vi "Test Read and Move.vi"(7 "Stop Button":bool, 10 "Auto Feed Control":T1) -> ()   [LabVIEW 2013]
doc: "This VI tests reading positions from all three axes simultaneously, and sending move commands to the\naxes using the NI Motion Assistant Move Hander."
uses:
  <vilib>/MotionAssistant/MotionAssistant.llb/Move Constraints.ctl
  <vilib>/MotionAssistant/MotionAssistant.llb/Velocity Profile Type Enum.ctl
  Controls/axis_indicator_cluster.ctl
  Controls/auto_feed_control_cluster.ctl
  <vilib>/MotionAssistant/MotionAssistant.llb/Straight Line Move Properties.ctl
  <vilib>/MotionAssistant/MotionAssistant.llb/Straight Line Dimension Enum.ctl
  <vilib>/MotionAssistant/MotionAssistant.llb/Straight Line Move Mode Enum.ctl
  <vilib>/MotionAssistant/MotionAssistant.llb/Coordinate Point.ctl
  Controls/PWM_data_cluster.ctl
  Controls/table_axis_enum.ctl
  Controls/PWM_state_enum.ctl
  <vilib>/MotionAssistant/MotionAssistant.llb/Profile Calculation Constraint.ctl
  <vilib>/MotionAssistant/MotionAssistant.llb/Array Constraints Spec Type Enum.ctl
  <vilib>/MotionAssistant/MotionAssistant.llb/Move Profile Enum.ctl
  <vilib>/MotionAssistant/MotionAssistant.llb/Open Straight Line Move Handle.vi
  <vilib>/MotionAssistant/MotionAssistant.llb/Close Straight Line Move Handle.vi
  <vilib>/MotionAssistant/MotionAssistant.llb/Set Straight Line Move Properties.vi
  <vilib>/MotionAssistant/MotionAssistant.llb/Get Straight Line Move Profile.vi
panel:
  out "Axis Inds.":T2 caption="Axis Indicators"
  in  "Move Constraints":T3={"Velocity Profile Type"=enum."S Curve", "Max Velocity"=2.0, "Max Acceleration"=1.0, "Max Deceleration"=1.0, "Max Jerk"=2.0, "Initial Velocity"=0.0, "Final Velocity"=0.0} {"Final Velocity" format="%#.6g"; "Initial Velocity" format="%#.6g"; "Max Jerk" format="%#.6g"; "Max Deceleration" format="%#.6g"; "Max Acceleration" format="%#.6g"; "Max Velocity" format="%#.6g"}
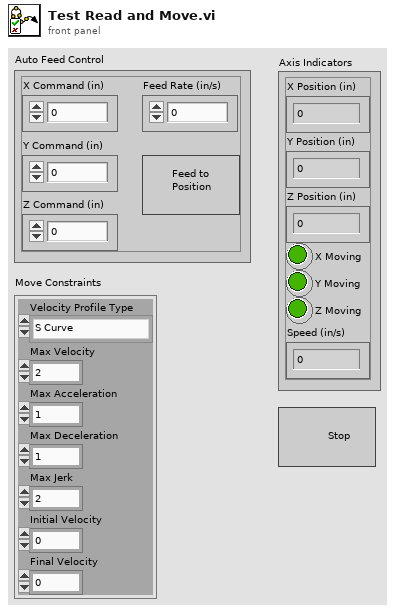
[diagram p1: front panel]
types:
  T1 = typedef "auto_feed_control_cluster.ctl" = cluster{"Feed Rate (in/s)":dbl, "X Command (in)":dbl, "Y Command (in)":dbl, "Z Command (in)":dbl, "feed to pos":bool}
  T2 = typedef "axis_indicator_cluster.ctl" = cluster{"X Position (in)":dbl, "Y Position (in)":dbl, "Z Position (in)":dbl, "X Moving":bool, "Y Moving":bool, "Z Moving":bool, "Speed (in/s)":dbl}
  T3 = typedef "Move Constraints.ctl" = cluster{"Velocity Profile Type":T4, "Max Velocity":dbl, "Max Acceleration":dbl, "Max Deceleration":dbl, "Max Jerk":dbl, "Initial Velocity":dbl, "Final Velocity":dbl}
  T4 = typedef "Velocity Profile Type Enum.ctl" = enum32{"Trapezoidal", "S Curve"}
  T5 = typedef "PWM_data_cluster.ctl" = cluster{"frequency":dbl, "Duty Cycle (%)":dbl, "Axis Enum":T6, "Function Enum":T7}
  T6 = typedef "table_axis_enum.ctl" = enum16{"X-axis", "Y-axis", "Z-axis", "W-axis"}
  T7 = typedef "PWM_state_enum.ctl" = enum16{"Initialize", "SetAxisSpeed", "StopAxis", "StopAll", "Shutdown"}
  T8 = typedef "Straight Line Move Properties.ctl" = cluster{"Dimension":T9, "Move Mode":T10, "Position Mode - End Point":T11, "Velocity Mode - Travel Time (sec)":dbl}
  T9 = typedef "Straight Line Dimension Enum.ctl" = enum16{"1-Dimension", "2-Dimension", "3-Dimension"}
  T10 = typedef "Straight Line Move Mode Enum.ctl" = enum32{" Position Mode", "Velocity Mode"}
  T11 = typedef "Coordinate Point.ctl" = cluster{"X":dbl, "Y":dbl, "Z":dbl}
  T12 = cluster{"Straight Line Move Properties":T8, "Start Point":T11}
  T13 = typedef "Straight Line Move Handle.ctl" = cluster{"Straight Line Move Enum":T14, "Move Handle":i32}
  T14 = typedef "Straight Line Move Enum.ctl" = enum16{"Straight Line Move"}
  T15 = typedef "Move Profile Enum.ctl" = enum16{"Velocity Profile", "Acceleration Profile", "Position Profile"}
  T16 = typedef "Profile Calculation Constraint.ctl" = cluster{"Constraint Type":T17, "Constraint Value":dbl}
  T17 = typedef "Array Constraints Spec Type Enum.ctl" = enum16{"Array Size", "Sampling Time"}
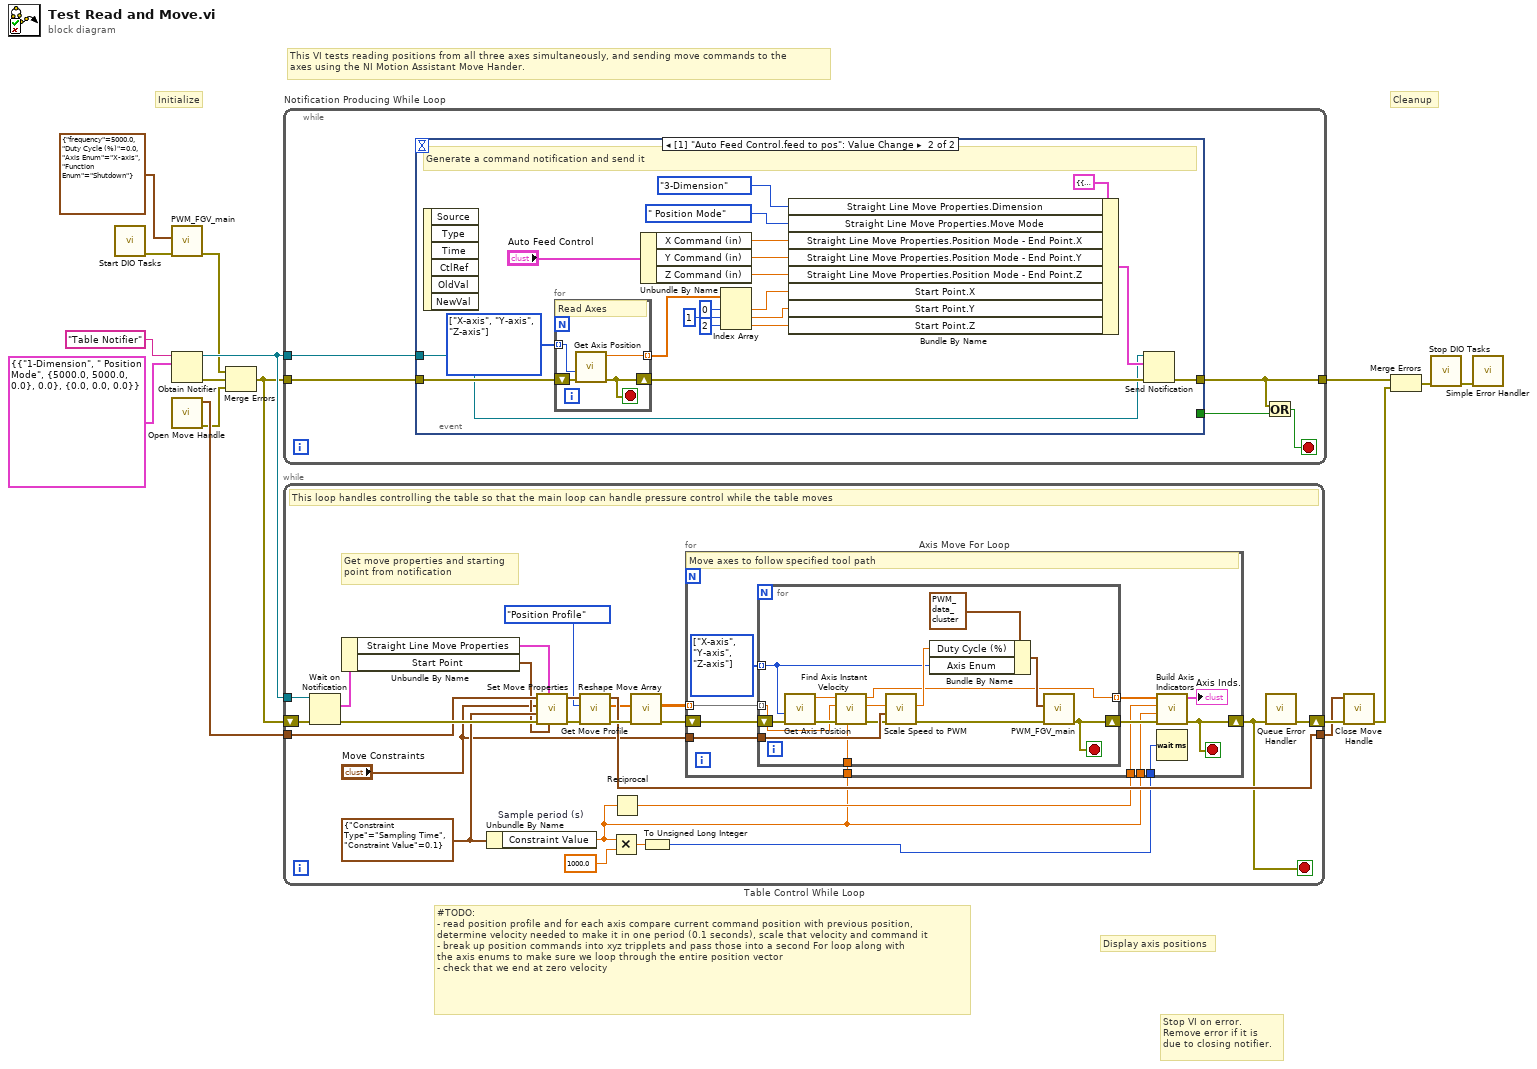
[diagram p0: block diagram]
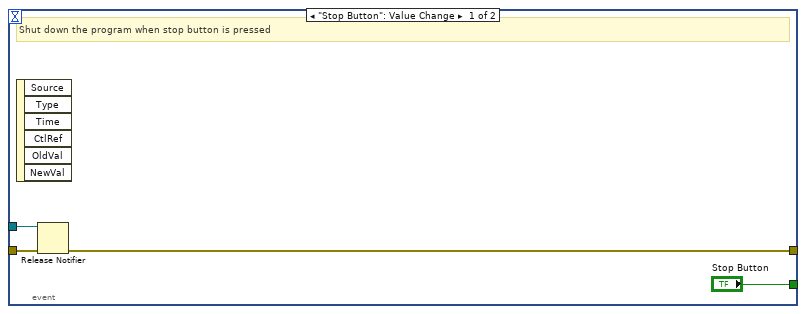
[diagram p2: hidden frame]
diagram:
  # "Stop VI on error.\nRemove error if it is\ndue to closing notifier."
  # "Display axis positions"
  # "#TODO:\n- read position profile and for each axis compare current command position with previous position,\ndetermine velocity needed to make it in one period (0.1 seconds), scale that velocity and command it\n- break up position commands into xyz tripplets and pass those into a second For loop along with\nthe axis enums to make sure we loop through the entire position vector\n- check that we end at zero velocity"
  # "Initialize"
  # "Cleanup"
  # "This VI tests reading positions from all three axes simultaneously, and sending move commands to the\naxes using the NI Motion Assistant Move Hander."
  n1 = call "Start DIO Tasks.vi"() -> ("error out"=w3:errorcluster)  [unwired: 11 in]
  n2 = call "PWM_FGV_main.vi"("Error In"=w3, "PWM FGV Data"=T5 {"frequency"=5000.0, "Duty Cycle (%)"=0.0, "Axis Enum"=enum."X-axis", "Function Enum"=enum."Shutdown"}) -> ("Error Out"=w8:errorcluster)  [unwired: 9 in]
  n3 = Obtain Notifier(name (unnamed)="Table Notifier", notification data type=T12 {"Straight Line Move Properties"={"Dimension"=enum."1-Dimension", "Move Mode"=enum." Position Mode", "Position Mode - End Point"={"X"=5000.0, "Y"=5000.0, "Z"=0.0}, "Velocity Mode - Travel Time (sec)"=0.0}, "Start Point"={"X"=0.0, "Y"=0.0, "Z"=0.0}}) -> (notifier out=w13:refnum<notifier>, error out=w12:errorcluster)  [unwired: 2 in, 1 out]
  n4 = call-poly <vilib>:"Open Move Handle.vi"() -> ("error out"=w11:errorcluster, "Straight Line Move Handle"=w16:T13)  [unwired: 9 in]
  n5 = Merge Errors(w8, w12, w11) -> (w10:errorcluster)
  n6 = while "Notification Producing While Loop" {
    tunnel: w13 -> [w17]
    tunnel: w10 -> [w18]
    tunnel: [w20] -> w4
    stop <- w21 stop-if-true
    n7 = event shown="[1] \"Auto Feed Control.feed to pos\": Value Change" {
      selector: _ -> [_ _]
      dyn-events: _ -> [_ _]
      timeout: _ -> [_ _]
      tunnel: ["Stop Button" _] -> w19
      tunnel: [w24 w45] -> w20
      tunnel: w18 -> [w23 w29]
      tunnel: w17 -> [w22 w28]
      event "Stop Button": Value Change {
        # "Shut down the program when stop button is pressed"
        n8 = event-data() -> ()  [unwired: 1 in, 6 out]
        n9 = Release Notifier(notifier=w22, error in (no error)=w23) -> (error out=w24:errorcluster)  [unwired: 1 in, 2 out]
      }
      event Value Change {
        w38 = T6[] [enum."X-axis", enum."Y-axis", enum."Z-axis"] items=["X-axis", "Y-axis", "Z-axis", "W-axis"]
        # "Generate a command notification and send it"
        n10 = event-data() -> ()  [unwired: 1 in, 6 out]
        n11 = for "Read Axes" {
          shift-right: [w48] -> w39
          shift-left: w29 -> [w49]
          tunnel: w38 -> [w47] mode=indexing
          tunnel: [w46] -> w37 mode=indexing
          stop <- w48 stop-if-true
          # "Read Axes"
          n12 = call "Get Axis Position.vi"("Error In"=w49, "Axis Enum"=w47) -> ("Error Out"=w48:errorcluster, "Axis Inches"=w46:dbl)  [unwired: 6 in, 2 out]
        }
        n13 = Unbundle By Name("Auto Feed Control") -> ("X Command (in)"=w42:dbl, "Y Command (in)"=w41:dbl, "Z Command (in)"=w40:dbl)
        n14 = Index Array(array=w37, index #1=0 ("index"), index #2=1 ("index"), index #3=2 ("index")) -> (element #1=w36:dbl, element #2=w34:dbl, element #3=w35:dbl)
        n15 = Bundle By Name(cluster=T12 {"Straight Line Move Properties"={"Dimension"=enum."1-Dimension", "Move Mode"=enum." Position Mode", "Position Mode - End Point"={"X"=0.0, "Y"=0.0, "Z"=0.0}, "Velocity Mode - Travel Time (sec)"=0.0}, "Start Point"={"X"=0.0, "Y"=0.0, "Z"=0.0}} ("notification"), "Straight Line Move Properties.Dimension"=Straight_Line_Dimension_Enum."3-Dimension", "Straight Line Move Properties.Move Mode"=Straight_Line_Move_Mode_Enum." Position Mode", "Straight Line Move Properties.Position Mode - End Point.X"=w42, "Straight Line Move Properties.Position Mode - End Point.Y"=w41, "Straight Line Move Properties.Position Mode - End Point.Z"=w40, "Start Point.X"=w36, "Start Point.Y"=w34, "Start Point.Z"=w35) -> (w30:T12)
        n16 = Send Notification(notification=w30, notifier=w28, error in (no error)=w39) -> (error out=w45:errorcluster)  [unwired: 1 out]
      }
    }
    n17 = Or(x=w20, y=w19) -> (x .or. y?=w21:bool)
  }
  n18 = while "Table Control While Loop" {
    shift-right: [w72] -> w7
    shift-left: w10 -> [w71]
    tunnel: w13 -> [w70]
    tunnel: w16 -> [w65]
    tunnel: [w57] -> w5
    stop <- w52 stop-if-true
    w63 = T16 {"Constraint Type"=enum."Sampling Time", "Constraint Value"=0.1} ("Profile Calculation Constraint")
    # "Get move properties and starting\npoint from notification"
    # "This loop handles controlling the table so that the main loop can handle pressure control while the table moves"
    n19 = Wait on Notification(notifier=w70, error in (no error)=w71) -> (notification=w60:T12, error out=w66:errorcluster)  [unwired: 2 in, 2 out]
    n20 = Unbundle By Name(w60) -> ("Straight Line Move Properties"=w59:T8, "Start Point"=w58:T11)
    n21 = Unbundle By Name "Sample period (s)"(w63) -> ("Constraint Value"=w54:dbl)
    n22 = call-poly <vilib>:"Set Move Properties.vi"("Start Point"=w58, "Straight Line Move Properties"=w59, "error in"=w66, "Profile Calculation Constraint"=w63, "Move Constraints"="Move Constraints", "Straight Line Move Handle In"=w65) -> ("error out"=w69:errorcluster, "Straight Line Move Handle Out"=w68:T13)  [unwired: 3 in]
    n23 = call-poly <vilib>:"Get Move Profile.vi"("error in"=w69, "Profile Type"=Move_Profile_Enum."Position Profile", "Straight Line Move Handle In"=w68) -> ("error out"=w67:errorcluster, "Profile"=w51:dbl[], "Straight Line Move Handle Out"=w57:T13)  [unwired: 3 in, 2 out]
    n24 = Multiply(x=w54, y=1000.0) -> (x*y=w62:dbl)
    n25 = Reciprocal(x=w54) -> (1/x=w55:dbl)
    n26 = call "Reshape Move Array.vi"("Profile in"=w51) -> ("Profile out"=w50:dbl[][])  [unwired: 10 in]
    n27 = To Unsigned Long Integer(number=w62) -> (unsigned 32bit integer=w53:u32)
    n28 = for "Axis Move For Loop" {
      shift-right: [w80] -> w52
      shift-left: w67 -> [w83]
      tunnel: "Move Constraints" -> [w84]
      tunnel: w50 -> [w82] mode=indexing
      tunnel: w54 -> [w81]
      tunnel: w55 -> [w75]
      tunnel: w54 -> [w76]
      tunnel: w53 -> [w77]
      stop <- w80 stop-if-true
      w74 = T6[] [enum."X-axis", enum."Y-axis", enum."Z-axis"] items=["X-axis", "Y-axis", "Z-axis", "W-axis"]
      # "Move axes to follow specified tool path"
      n29 = for {
        tunnel: w84 -> [w99]
        tunnel: w82 -> [w90] mode=indexing
        tunnel: w81 -> [w88]
        shift-right: [w86] -> w79
        shift-left: w83 -> [w95]
        tunnel: w74 -> [w87] mode=indexing
        tunnel: [w85] -> w73 mode=indexing
        stop <- w86 stop-if-true
        n30 = call "Get Axis Position.vi"("Error In"=w95, "Axis Enum"=w87) -> ("Error Out"=w93:errorcluster, "Axis Inches"=w92:dbl)  [unwired: 6 in, 2 out]
        n31 = call "Find Axis Instant Velocity.vi"("Sample Period"=w88, "Error In"=w93, "Desired Position"=w90, "Current Position"=w92) -> ("Error Out"=w89:errorcluster, "Axis Velocity"=w91:dbl, "Current Position out"=w85:dbl)  [unwired: 5 in]
        n32 = call "Scale Speed to PWM.vi"("Error In"=w89, "Move Constraints"=w99, "Desired Speed (in/s)"=w91) -> ("Error Out"=w94:errorcluster, "Motor Duty Cycle"=w96:dbl)  [unwired: 7 in]
        n33 = Bundle By Name(cluster=T5 {"frequency"=5000.0, "Duty Cycle (%)"=0.0, "Axis Enum"=enum."X-axis", "Function Enum"=enum."Shutdown"} ("PWM FGV Data"), "Duty Cycle (%)"=w96, "Axis Enum"=w87) -> (w97:T5)
        n34 = call "PWM_FGV_main.vi"("Error In"=w94, "PWM FGV Data"=w97) -> ("Error Out"=w86:errorcluster)  [unwired: 9 in]
      }
      n35 = call "Build Axis Indicators.vi"("Error In"=w79, "Sample Period"=w76, "Sample Freq."=w75, "Axis Pos."=w73) -> ("Error Out"=w80:errorcluster, "Axis Inds. out"=→"Axis Inds.":T2)  [unwired: 6 in]
      n36 = Wait (ms)(milliseconds to wait=w77) -> ()  [unwired: 1 out]
    }
    n37 = call "Queue Error Handler.vi"("Error In"=w52) -> ("Error Out"=w72:errorcluster)  [unwired: 10 in]
  }
  n38 = call-poly <vilib>:"Close Move Handle.vi"("error in"=w7, "Straight Line Move Handle"=w5) -> ("error out"=w6:errorcluster)  [unwired: 8 in]
  n39 = Merge Errors(w4, w6) -> (w2:errorcluster)
  n40 = call "Stop DIO Tasks.vi"("Error In"=w2) -> ("error out"=w1:errorcluster)  [unwired: 10 in]
  n41 = call <vilib>:"Simple Error Handler.vi"("error in (no error)"=w1) -> ()  [unwired: 4 in, 5 out]
